vi "Configure Acquisition.vi"(0 "RedPitaya connection in":refnum<k5>, 1 "Decimation/Sampling Rate":string(combo), 2 "Sampling Rate":string(combo)="1_9kHz", 3 "Decimation":u32(ring) items=["65536"=65536, "8192"=8192, "1024"=1024, "64"=64, "8"=8, "1"=1], 4 "Averaging":enum16{"None", "AVG ON", "AVG OFF"}(ring), 5 "error in":errorcluster, 12 "timeout ms (2000)":i32=2000) -> (14 "RedPitaya connection out":refnum<k5>, 19 "error out":errorcluster)   [LabVIEW 2010, in "RedPitaya.lvlib"]
doc: "Configures the propertise of acquisition. To set acquisition decimation or sampling rate first select which you want to set by input <b>Decimation/Sampling Rate</b>.\n\nCall this VI for each channel you want to configure waveform acquisition settings."
uses:
  RedPitaya.lvlib
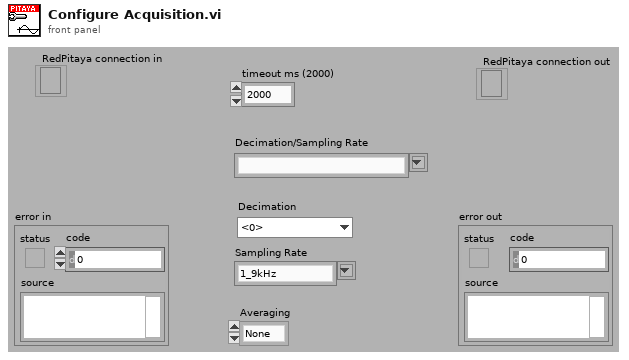
[diagram p1: front panel]
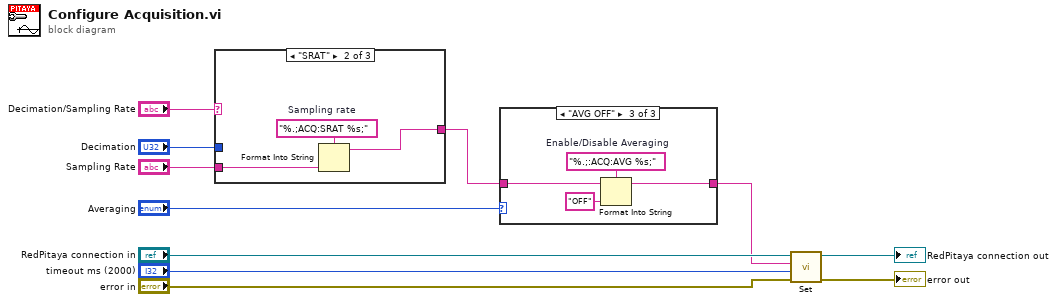
[diagram p0: block diagram]
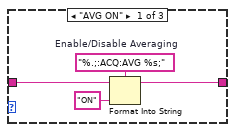
[diagram p2: hidden frame]
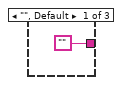
[diagram p4: hidden frame]
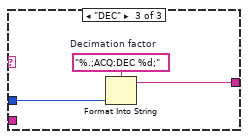
[diagram p5: hidden frame]
diagram:
  n1 = case shown="\"SRAT\"" "Decimation/Sampling Rate" {
    tunnel: ["" w15 w17] -> w11
    tunnel: "Sampling Rate" -> [_ w14 _]
    tunnel: "Decimation" -> [_ _ w16]
    frame "", Default {
    }
    frame "SRAT" {
      w13 = "%.;ACQ:SRAT %s;"  # Sampling rate
      n2 = Format Into String(format string=w13, w14) -> (resulting string=w15:string)  [unwired: 2 in, 1 out]
    }
    frame "DEC" {
      w18 = "%.;ACQ:DEC %d;"  # Decimation factor
      n3 = Format Into String(format string=w18, w16) -> (resulting string=w17:string)  [unwired: 2 in, 1 out]
    }
  }
  n4 = case shown="\"AVG OFF\"" "Averaging" {
    tunnel: [w22 w23 w27] -> w6
    tunnel: w11 -> [w21 w23 w26]
    frame "AVG ON" {
      w20 = "%.;:ACQ:AVG %s;"  # Enable/Disable Averaging
      n5 = Format Into String(format string=w20, initial string=w21, "ON") -> (resulting string=w22:string)  [unwired: 1 in, 1 out]
    }
    frame "None", Default {
    }
    frame "AVG OFF" {
      w25 = "%.;:ACQ:AVG %s;"  # Enable/Disable Averaging
      n6 = Format Into String(format string=w25, initial string=w26, "OFF") -> (resulting string=w27:string)  [unwired: 1 in, 1 out]
    }
  }
  n7 = call "Set.vi"("error in"="error in", "timeout ms (2000)"="timeout ms (2000)", "SCPI Message"=w6, "RedPitaya connection in"="RedPitaya connection in") -> ("error out"=→"error out":errorcluster, "RedPitaya connection out"=→"RedPitaya connection out":refnum<k5>)  [unwired: 5 in, 1 out]
